vi "SetTriggerHW.vi"(8 "error in (no error)":errorcluster, 11 "BME_DG_G05 in":refnum<class "BME_DG_G05.lvclass">) -> (0 "error out":errorcluster, 3 "BME_DG_G05 out":refnum<class "BME_DG_G05.lvclass">)   [LabVIEW 2009, in "POLARIS BME DG.lvlib" / "BME_DG_G05.lvclass"]
uses:
  BME_DG_G05.lvclass
  BME_DG_Base/BME_DG_Base.lvclass
  BME_DG_G05.lvclass/BME_DG_G05.ctl
  POLARIS BME DG.lvlib
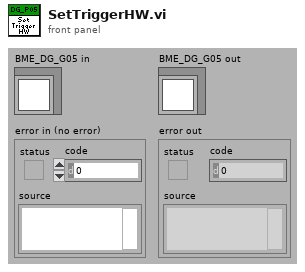
[diagram p1: front panel]
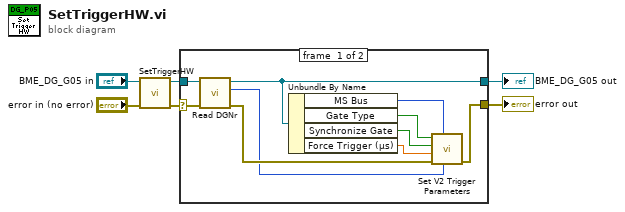
[diagram p0: block diagram]
diagram:
  n1 = call-parent "SetTriggerHW.vi"("error in (no error)"="error in (no error)", "BME_DG_Base in"="BME_DG_G05 in") -> ("error out"=w3:errorcluster, "BME_DG_Base out"=w6:refnum<class "BME_DG_G05.lvclass">)  [unwired: 8 in]
  n2 = case shown="No Error" w3 {
    selector: w3 -> [w9 w17]
    tunnel: w6 -> [w11 w18]
    tunnel: [w10 w18] -> w2
    tunnel: [w16 w17] -> w1
    frame #0 {
      n3 = call-dynamic "Read DGNr.vi"("error in (no error)"=w9, "BME_DG_Base in"=w11) -> ("error out"=w8:errorcluster, "DGNr"=w7:i32, "BME_DG_Base out"=w10:refnum<class "BME_DG_G05.lvclass">)  [unwired: 7 in]
      n4 = Unbundle By Name(w10) -> ("MS Bus"=w12:u32, "Gate Type"=w15:bool, "Synchronize Gate"=w14:bool, "Force Trigger (µs)"=w13:dbl)
      n5 = call "Set V2 Trigger Parameters.vi"("DG Number"=w7, "MS Bus"=w12, "error in (no error)"=w8, "Force Trigger (µs)"=w13, "Synchronize Gate"=w14, "Gate Type"=w15) -> ("error out"=w16:errorcluster)  [unwired: 5 in]
    }
    frame #1 {
    }
  }
  "BME_DG_G05 out" <- w2
  "error out" <- w1
